vi "Set JSON Config.vi"(8 "error in (no error)":errorcluster, 10 "<JSON>Config>":string, 11 "CFG Base in":refnum<class "CFG Base.lvclass">) -> (0 "error out":errorcluster, 3 "CFG Base out":refnum<class "CFG Base.lvclass">)   [LabVIEW 2023, in "HAL GOOP4.lvlib" / "CFG Base.lvclass"]
uses:
  CFG Base.lvclass
  CFG Base.lvclass/CFG Base.ctl
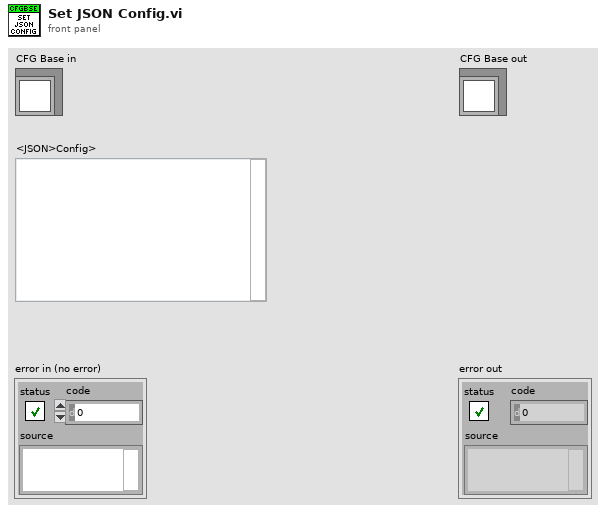
[diagram p1: front panel]
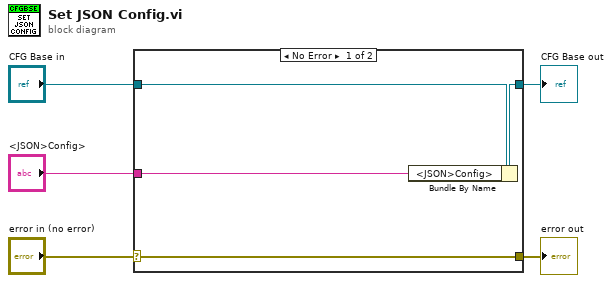
[diagram p0: block diagram]
diagram:
  n1 = case shown="No Error" "error in (no error)" {
    selector: "error in (no error)" -> [w9 w10]
    tunnel: [w9 w10] -> w4
    tunnel: [w7 w11] -> w2
    tunnel: "CFG Base in" -> [w8 w11]
    tunnel: "<JSON>Config>" -> [w6 _]
    frame No Error {
      n2 = Bundle By Name(cluster=w8, "<JSON>Config>"=w6) -> (w7:refnum<class "CFG Base.lvclass">)
    }
    frame Error {
    }
  }
  "error out" <- w4
  "CFG Base out" <- w2
